vi "EOL Manual Sunroof Control.vi"(7 "remote sense enabled":bool, 9 "DO Task":refnum<k21>, 10 "station name":string, 11 "station idx":i32=4) -> ()   [LabVIEW 2018]
uses:
  02.Type Def's/EOL Analog Input Control.ctl
  02.Type Def's/All Motions.ctl
  05.UserVI's/type defs/EOL Part Setup.ctl
  02.Type Def's/All Communication Types.ctl
  05.UserVI's/type defs/Communication with Motors.ctl
  05.UserVI's/type defs/RAP Signal Control.ctl
  05.UserVI's/type defs/EOL Motor Type.ctl
  02.Type Def's/All Switch Configuration Cluster.ctl
  05.UserVI's/type defs/EOL Global Digital Output Control.ctl
  05.UserVI's/type defs/EOL Global Digital Output Cluster Control.ctl
panel:
  out "Part Infos":T1[](array[typedef])
  in  "Exit":bool
  in  "Tab Control 3":enum32{"Select Program", "Sunroof Operation"}(tab)=enum."Sunroof Operation"
  in  "Part Type Selected":bool
  in  "Part Type":u16(ring) items=["CD701", "NU2", "A07", "B41", "B26", "B30", "J4U"]
  in  "sunroof 4":bool
  in  "sunroof 3":bool
  in  "sunroof 2":bool
  in  "sunroof":bool
  in  "Ignition":bool
  in  "Power":bool
  in  "Switch Output":bool
  out "Audit Graph":sgl[][](graph)
  in  "Analog Control":T6=enum."Motor Voltage"
  in  "Analog Control 2":T6=enum."Motor Current"
  in  "Analog Control 3":T6=enum."Switch A"
  in  "Color Box 10":u32(colorbox)=16860
  in  "Color Box 11":u32(colorbox)=16711680
  in  "Color Box 12":u32(colorbox)
  in  "Current Motion":T7=enum."Glass Slide Open"
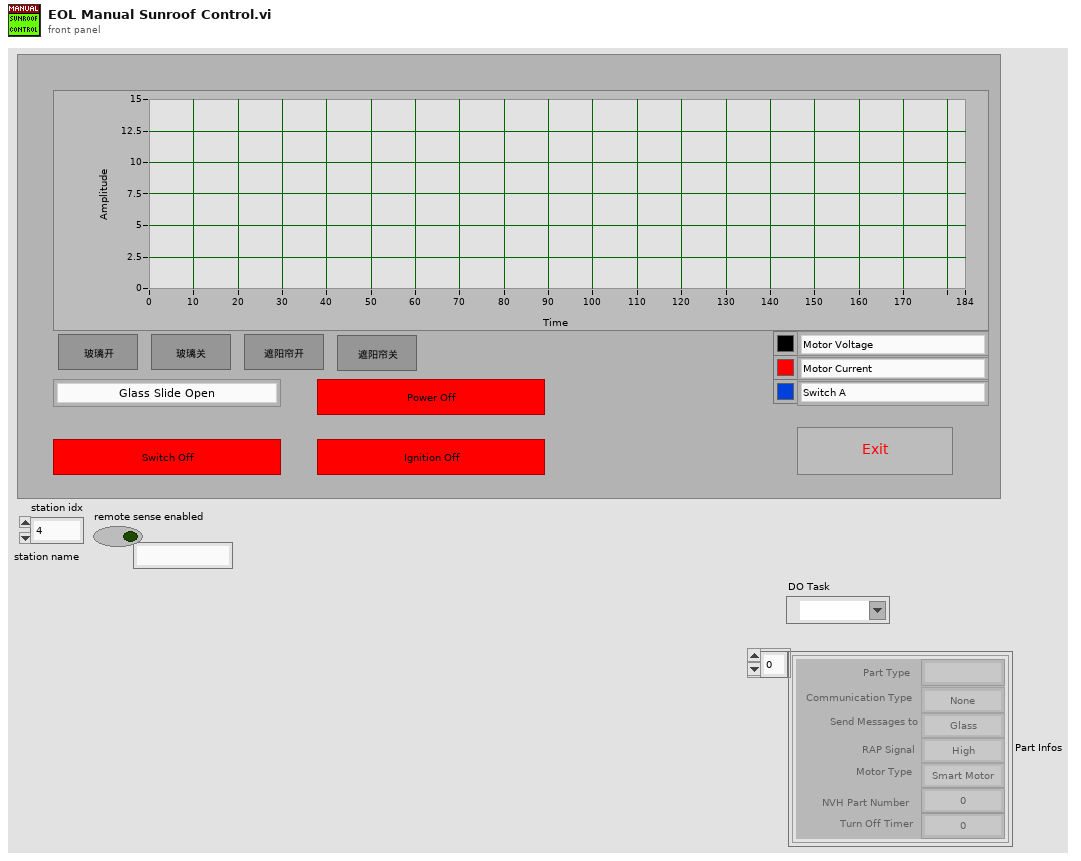
[diagram p1: front panel]
types:
  T1 = typedef "EOL Part Setup.ctl" = cluster{"Communication Type":T2, "Send Messages to":T3, "RAP Signal":T4, "Motor Type":T5, "NVH Part Number":u16, "Turn Off Timer":u16, "Part Type":string}
  T2 = typedef "All Communication Types.ctl" = enum16{"None", "CAN", "RS 232", "RS 232 LIN", "GM LIN", "SnT LIN", "K Line", "Robel CAN", "P42M-Continental", "Inalfa SCU LIN", "Spare 3"}
  T3 = typedef "Communication with Motors.ctl" = enum16{"Glass", "Rollo", "Both"}
  T4 = typedef "RAP Signal Control.ctl" = enum16{"High", "Low", "None"}
  T5 = typedef "EOL Motor Type.ctl" = enum16{"Smart Motor", "Sensor Motor"}
  T6 = typedef "EOL Analog Input Control.ctl" = enum16{"SW PS  Volage", "Switch A", "Switch B", "Switch C", "Motor Voltage", "Motor Current", "ATS"}
  T7 = typedef "All Motions.ctl" = enum16{"Glass Teach", "Glass Slide Open", "Glass Slide Close", "Glass Vent Open", "Glass Vent Close", "Sunshade Teach", "Sunshade Open", "Sunshade Close", "Idle", "Sunshade Open 2", "Sunshade Close 2", "Glass Slide Open Sunshade Open", "Glass Slide Open Sunshade Close", "Glass Slide Close Sunshade Open", "Glass Slide Close Sunshade Close", "Glass Vent Open Sunshade Open", "Glass Vent Open Sunshade Close", "Glass Vent Close Sunshade Open", "Glass Vent Close Sunshade Close", "Express Glass Slide Open", "Express Glass Slide Close", "Express Glass Vent Open", "Express Glass Vent Close", "Express Sunshade Open", "Express Sunshade Close", "Express Sunshade Open 2", "Express Sunshade Close 2", "Express Glass Slide Open Sunshade Open", "Express Glass Slide Open Sunshade Close", "Express Glass Slide Close Sunshade Open", "Express Glass Slide Close Sunshade Close", "Express Glass Vent Open Sunshade Open", "Express Glass Vent Open Sunshade Close", "Express Glass Vent Close Sunshade Open", "Express Glass Vent Close Sunshade Close", "Goto Position Glass", "Goto Position Sunshade", "Sunshade Teach 2"}
  T8 = typedef "All Switch Configuration Cluster.ctl" = cluster{"All Motions":T7, "A":bool[], "B":bool[], "C":bool[], "D":bool[], "A activation time (ms)":u32, "B activation time (ms)":u32, "C activation time (ms)":u32}
  T9 = cluster{"Part Type":string, "Switch Configuration":T8[]}
  T10 = enum16{"Init", "Write", "Write All", "Clear All", "Stop", "Read"}
  T11 = typedef "EOL Global Digital Output Control.ctl" = enum16{"Battery", "IGN High", "IGN Low", "LIN", "CAN", "Switch 1", "Switch 2", "Switch 3", "Switch 4", "Switch 5", "Switch 6", "Glass Analog Switch 1", "Glass Analog Switch 2", "Glass Analog Switch 3", "Glass Analog Switch 4", "Sunshade Analog Switch 1", "Sunshade Analog Switch 2", "Sunshade Analog Switch 3", "Sunshade Analog Switch 4", "Glass Motor Relay 1", "Glass Motor Relay 2", "Sunshade Motor Relay 1", "Sunshade Motor Relay 2"}
  T12 = typedef "EOL Global Digital Output Cluster Control.ctl" = cluster{"Status":bool, "Global DO Ch":T11}
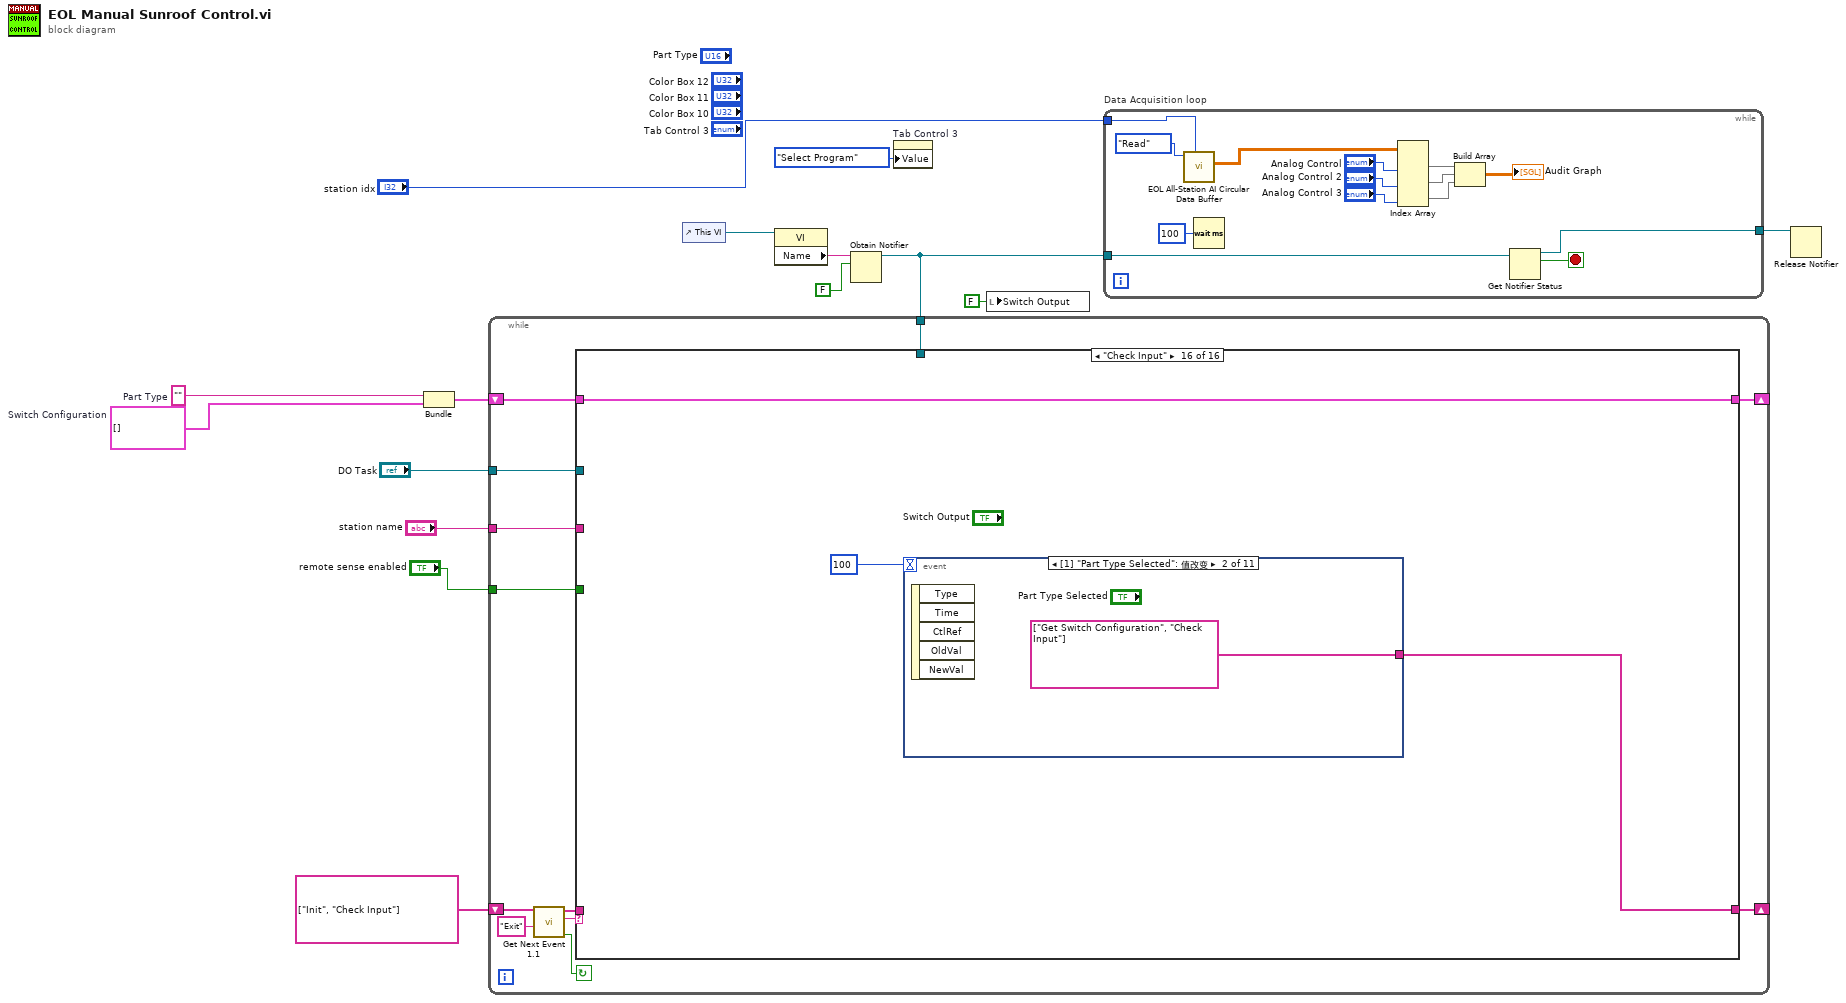
[diagram p0: block diagram]
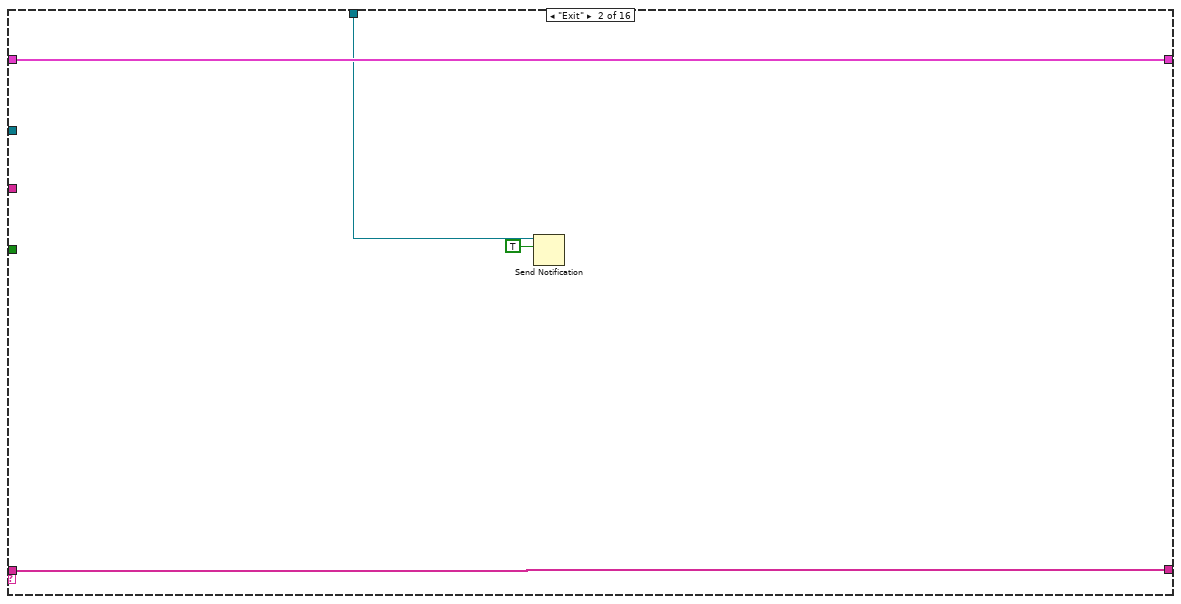
[diagram p3: hidden frame]
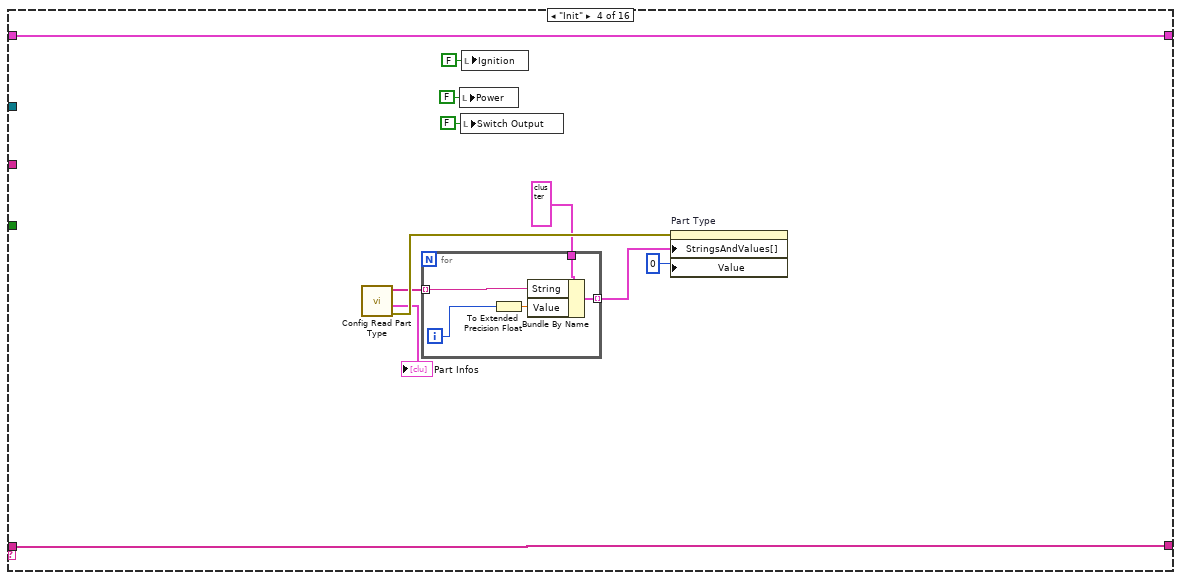
[diagram p5: hidden frame]
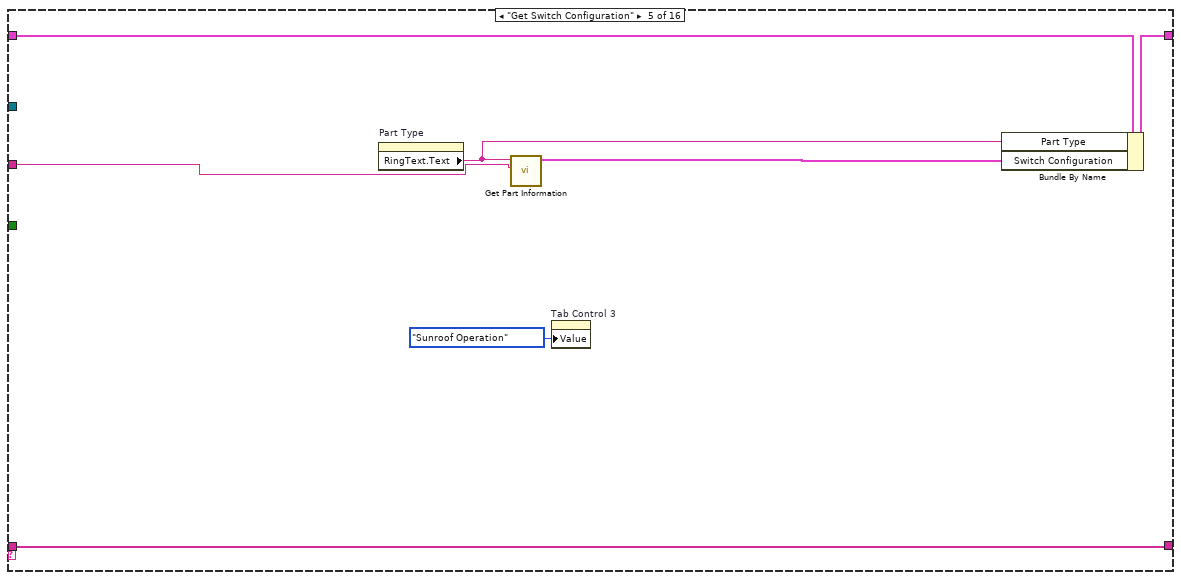
[diagram p6: hidden frame]
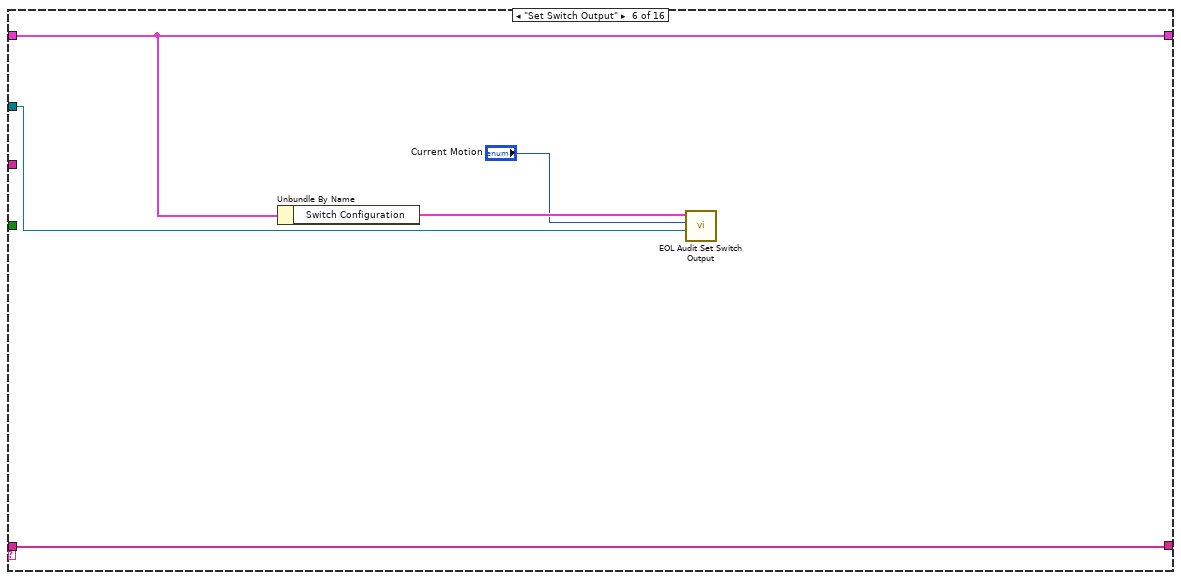
[diagram p7: hidden frame]
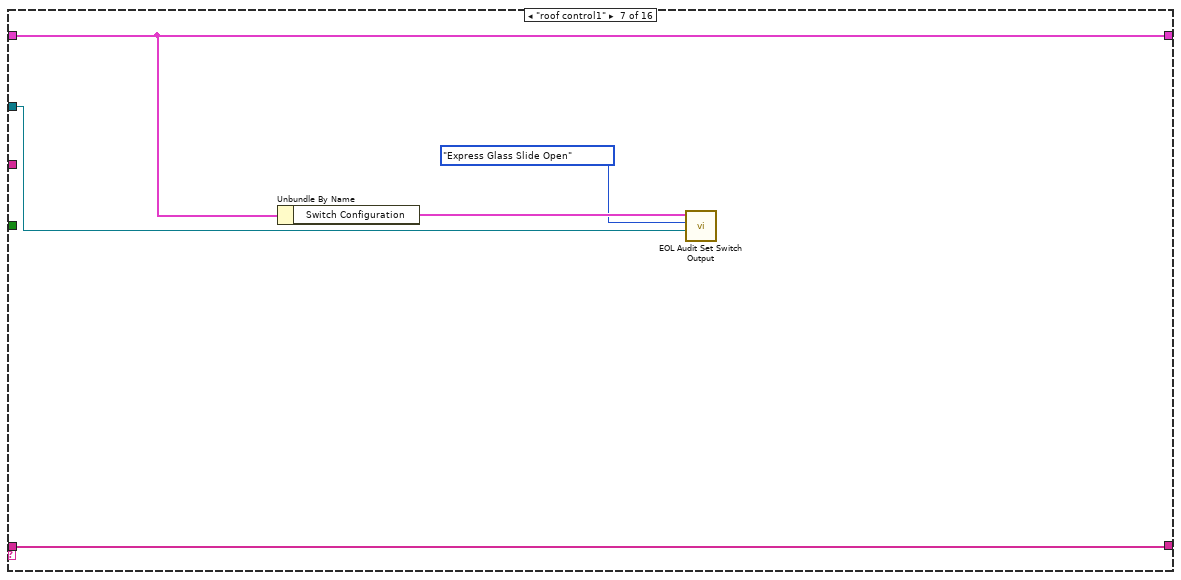
[diagram p8: hidden frame]
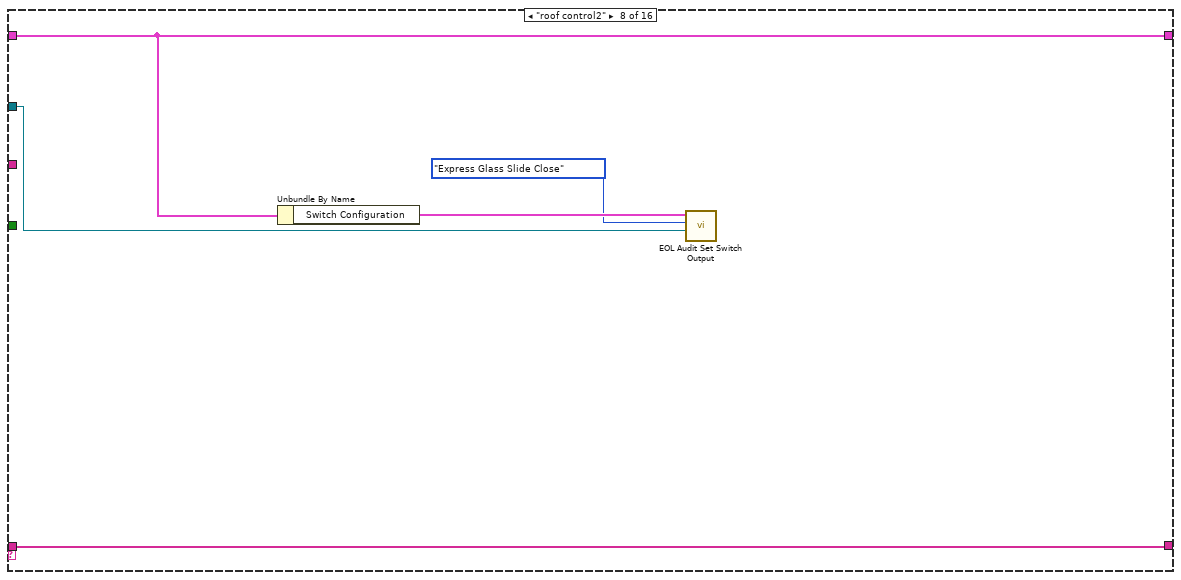
[diagram p9: hidden frame]
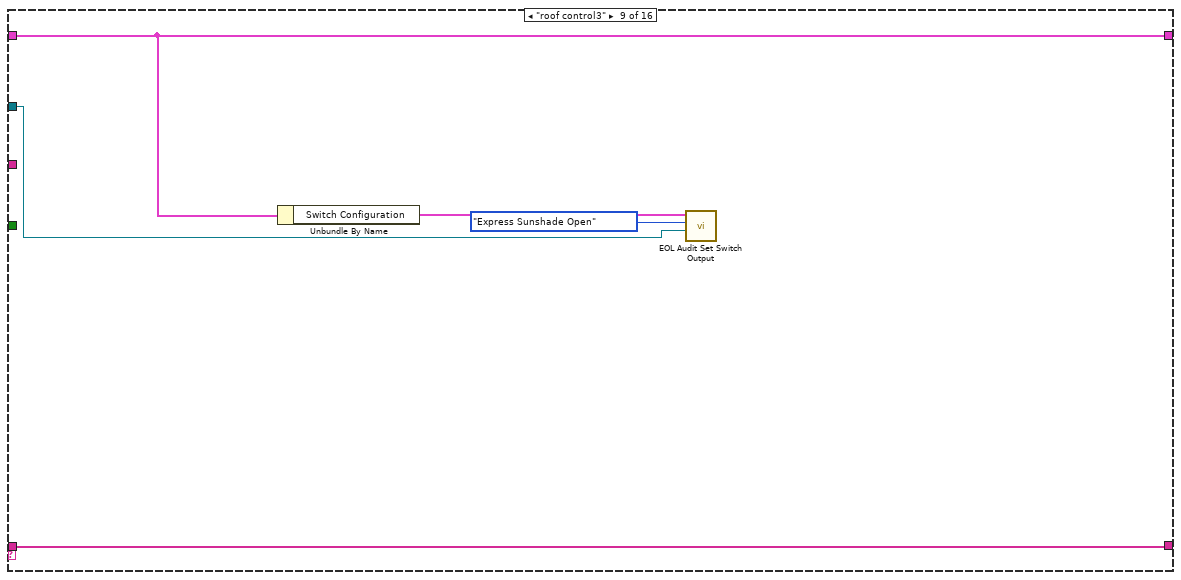
[diagram p10: hidden frame]
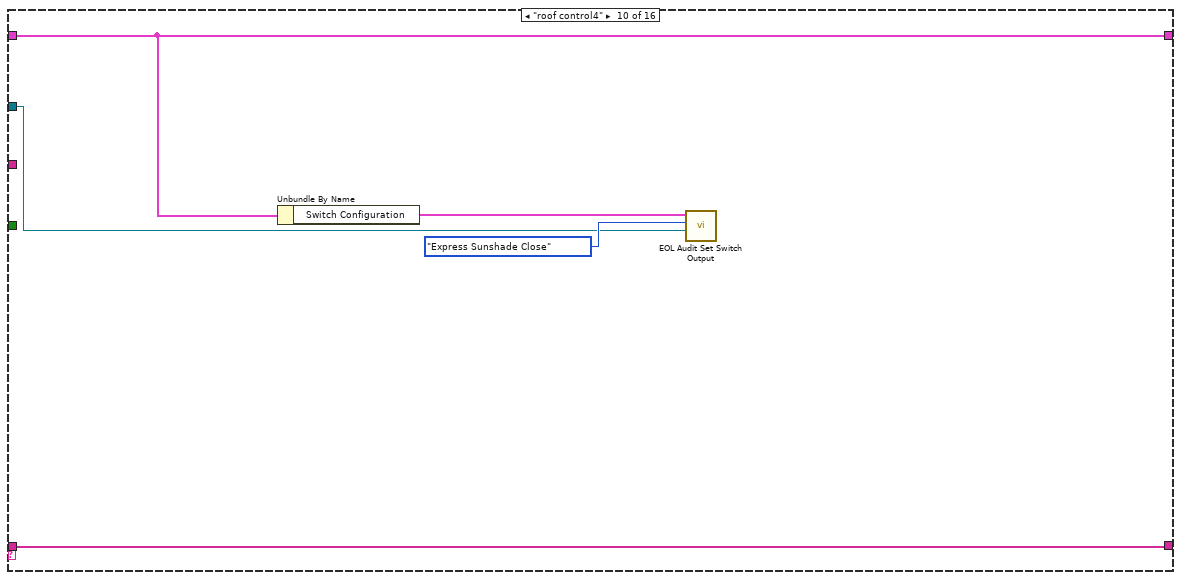
[diagram p11: hidden frame]
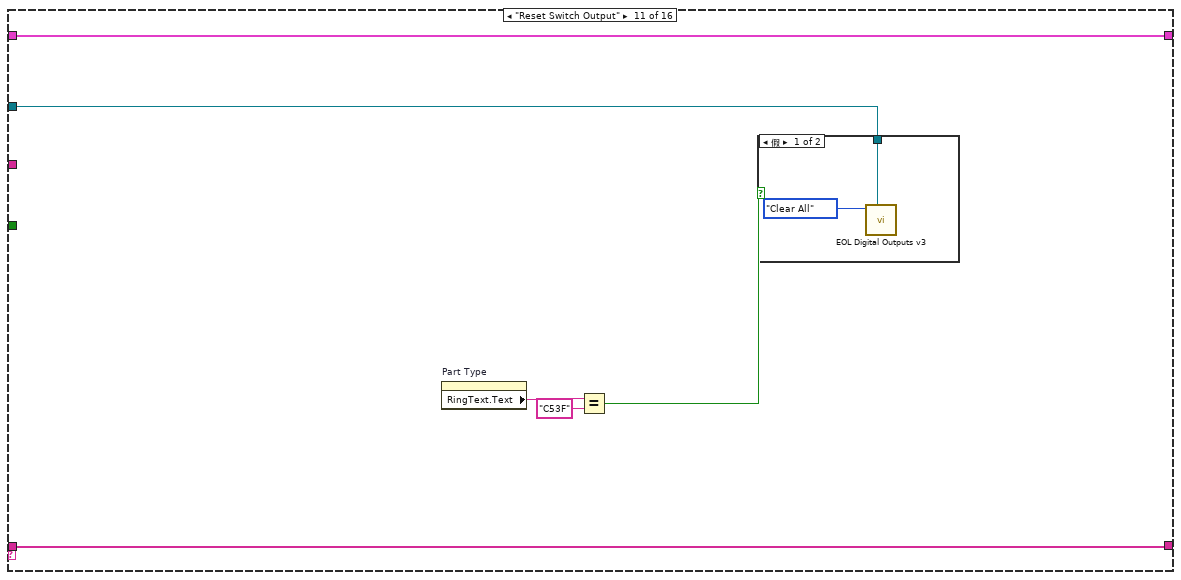
[diagram p12: hidden frame]
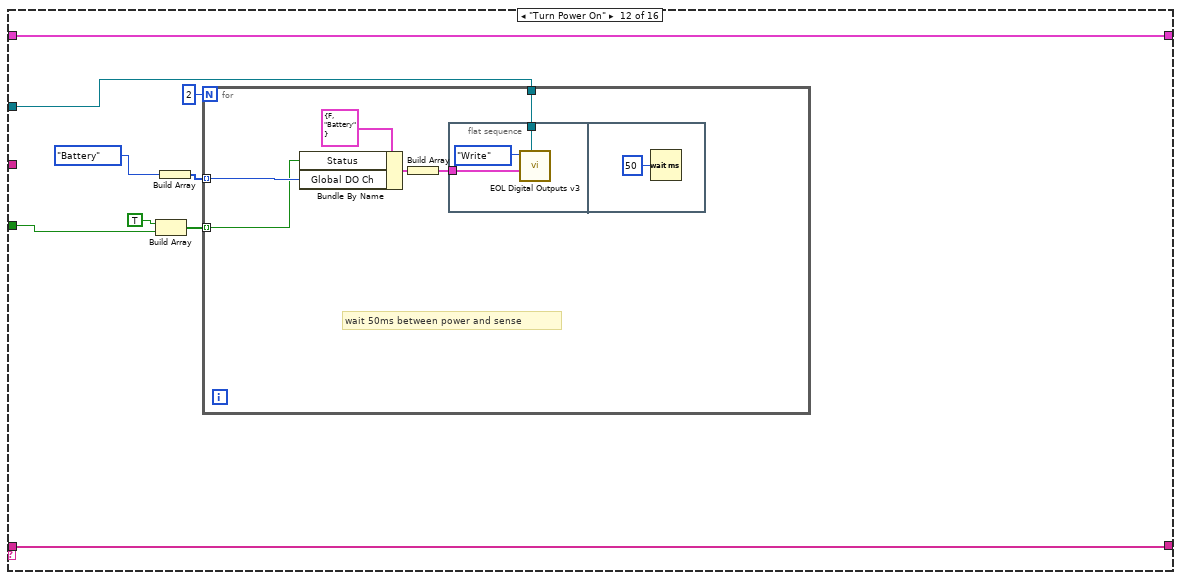
[diagram p14: hidden frame]
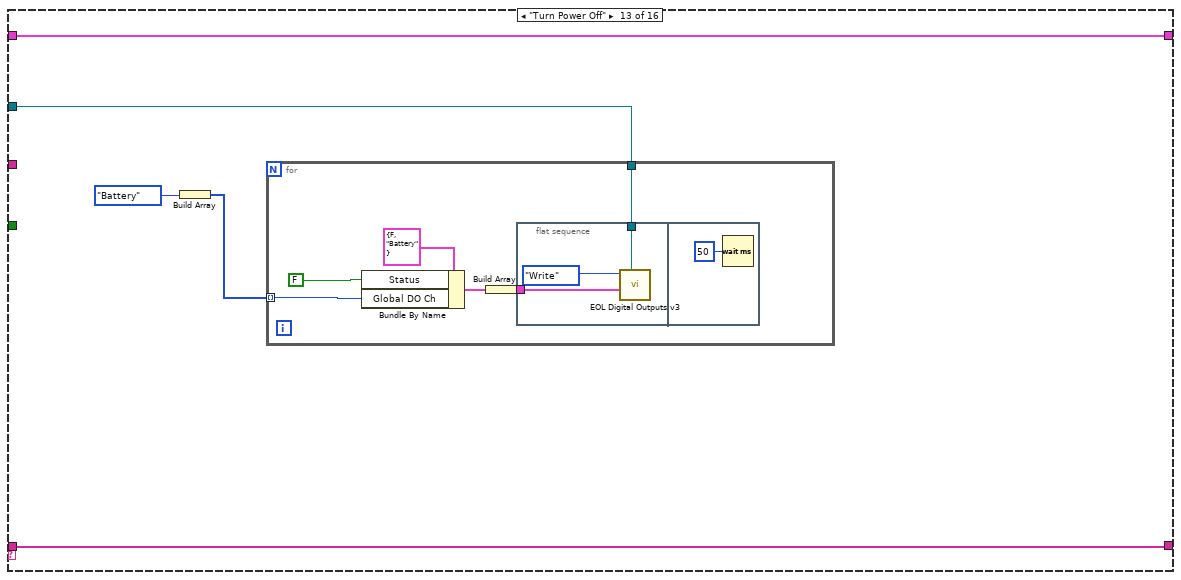
[diagram p15: hidden frame]
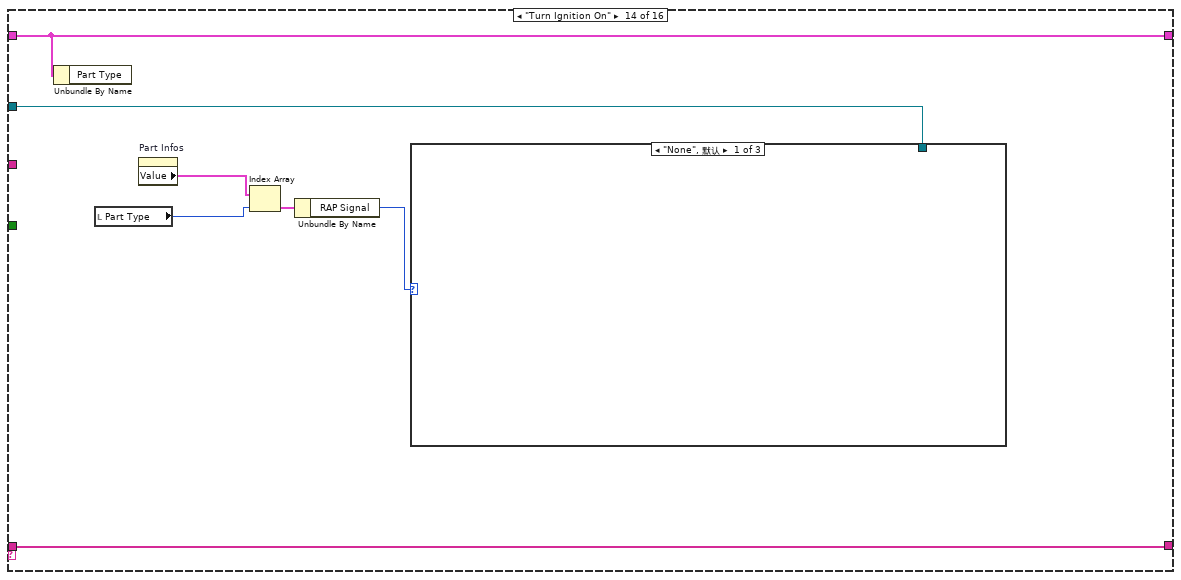
[diagram p16: hidden frame]
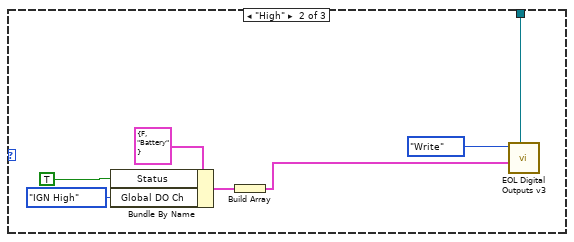
[diagram p17: hidden frame]
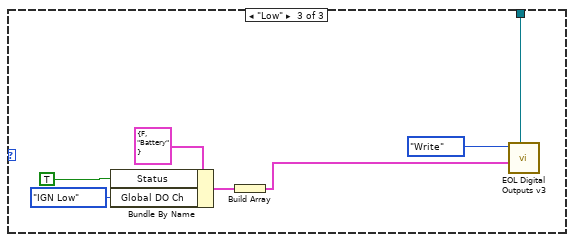
[diagram p18: hidden frame]
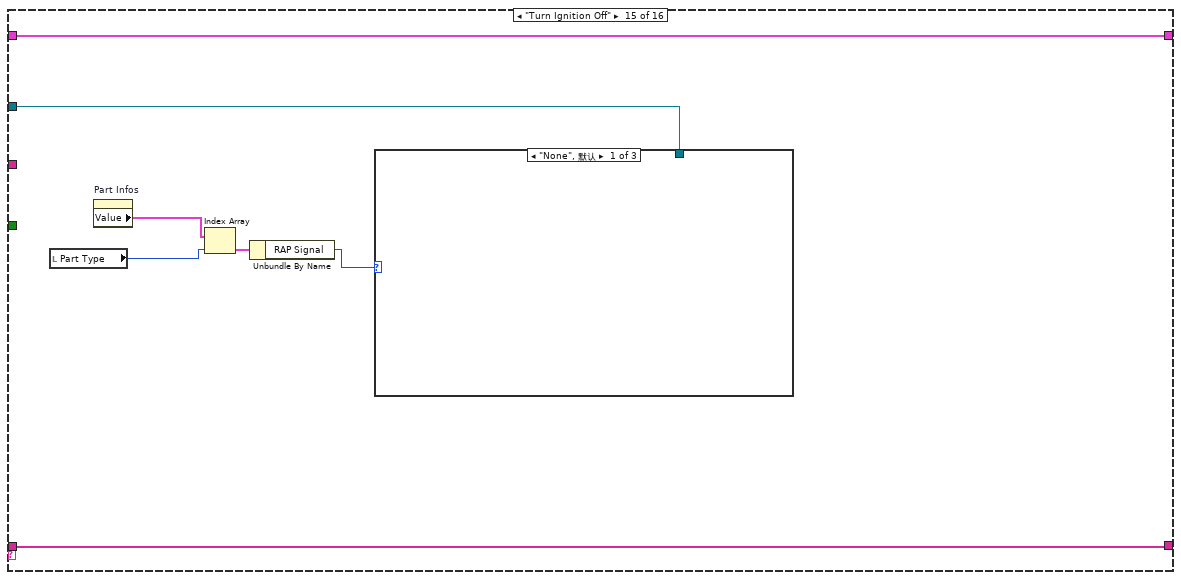
[diagram p19: hidden frame]
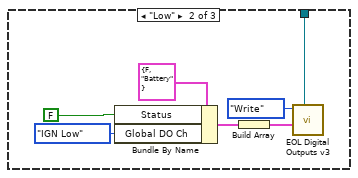
[diagram p20: hidden frame]
diagram:
  w12 = T8[] []  # Switch Configuration
  w14 = ""  # Part Type
  n1 = Bundle("Part Type"=w14, "Switch Configuration"=w12) -> (w15:T9)  [unwired: 1 in]
  n2 = control-ref of="This VI"() -> (w6:refnum<vi>)
  n3 = property class="VI"(reference=w6) -> ("Name"=w10:string)  [unwired: 1 in, 2 out]
  n4 = Obtain Notifier(name (unnamed)=w10, notification data type=FALSE) -> (notifier out=w8:refnum<notifier>)  [unwired: 2 in, 2 out]
  n5 = while {
    shift-right: [w25] -> _
    shift-left: string[] ["Init", "Check Input"] ("event queue out") -> [w24]
    shift-right: [w22] -> _
    shift-left: w15 -> [w23]
    tunnel: w8 -> [w19]
    tunnel: "station name" -> [w18]
    tunnel: "remote sense enabled" -> [w17]
    tunnel: "DO Task" -> [w16]
    stop <- w21 continue-if-true
    n6 = call "Get Next Event 1.1.vi"("Exit Event"="Exit", "event queue in"=w24) -> ("Condition (Exit:F)"=w21:bool, "next event"=w27:string, "event queue out"=w26:string[])  [unwired: 6 in, 1 out]
    n7 = case shown="\"Check Input\"" w27 {
      tunnel: w26 -> [w29 w33 w34 w46 w58 w63 w68 w73 w78 w83 w89 w99 w114 w132 w152 _]
      tunnel: [w29 w33 w34 w46 w58 w63 w68 w73 w78 w83 w89 w99 w114 w132 w152 w169] -> w25
      tunnel: w23 -> [w28 w32 w35 w45 w57 w62 w67 w72 w77 w82 w88 w100 w115 w130 w153 w170]
      tunnel: [w28 w32 w35 w45 w56 w62 w67 w72 w77 w82 w88 w100 w115 w130 w153 w170] -> w22
      tunnel: w19 -> [_ w31 _ _ _ _ _ _ _ _ _ _ _ _ _ _]
      tunnel: w18 -> [_ _ _ _ w52 _ _ _ _ _ _ _ _ _ _ _]
      tunnel: w17 -> [_ _ _ _ _ _ _ _ _ _ _ w96 _ _ _ _]
      tunnel: w16 -> [_ _ _ _ _ w59 w64 w69 w74 w79 w84 w92 w111 w131 w151 _]
      frame "Error", Default {
      }
      frame "Exit" {
        n8 = Send Notification(notification=TRUE, notifier=w31) -> ()  [unwired: 1 in, 2 out]
      }
      frame "Analog Data" {
      }
      frame "Init" {
        n9 = call "Config Read Part Type.vi"() -> ("Error Out"=w44:errorcluster, "Part Infos"=→"Part Infos":T1[], "Part Types"=w40:string[])  [unwired: 9 in]
        n10 = for {
          tunnel: cluster{"String":string, "Value":ext} {"String"="", "Value"=0.0} -> [w51]
          tunnel: w40 -> [w49] mode=indexing
          tunnel: [w48] -> w41 mode=indexing
          i -> [w47]
          n11 = To Extended Precision Float(1:w47) -> (0:w50:ext)
          n12 = Bundle By Name(cluster=w51, "String"=w49, "Value"=w50) -> (w48:cluster{"String":string, "Value":ext})
        }
        n13 = local write "Power"(FALSE ("Power")) -> ()
        n14 = local write "Switch Output"(FALSE ("Switch Output")) -> ()
        n15 = local write "Ignition"(FALSE ("Ignition")) -> ()
        n16 = property on="Part Type" class="Ring (strict)"(error in=w44, "StringsAndValues[]"=w41, "Value"=u16 0) -> ()  [unwired: 1 in, 2 out]
      }
      frame "Get Switch Configuration" {
        n17 = property on="Part Type" class="Ring (strict)"() -> ("RingText.Text"=w54:string)  [unwired: 2 in, 2 out]
        n18 = call "Get Part Information.vi"("station name"=w52, "Part Type"=w54) -> ("Switch Configuration"=w55:T8[])  [unwired: 1 in, 8 out]
        n19 = property on="Tab Control 3" class="TabCtl (strict)"("Value"=enum32{"Select Program", "Sunroof Operation"}."Sunroof Operation" ("Tab Control 3")) -> ()  [unwired: 2 in, 2 out]
        n20 = Bundle By Name(cluster=w57, "Part Type"=w54, "Switch Configuration"=w55) -> (w56:T9)
      }
      frame "Set Switch Output" {
        n21 = Unbundle By Name(w62) -> ("Switch Configuration"=w61:T8[])
        n22 = call "EOL Audit Set Switch Output.vi"("task/channels in"=w59, "Current Motion"="Current Motion", "Switch Output Array"=w61) -> ()  [unwired: 6 in, 3 out]
      }
      frame "roof control1" {
        n23 = Unbundle By Name(w67) -> ("Switch Configuration"=w66:T8[])
        n24 = call "EOL Audit Set Switch Output.vi"("task/channels in"=w64, "Current Motion"=All_Motions."Express Glass Slide Open", "Switch Output Array"=w66) -> ()  [unwired: 6 in, 3 out]
      }
      frame "roof control2" {
        n25 = Unbundle By Name(w72) -> ("Switch Configuration"=w71:T8[])
        n26 = call "EOL Audit Set Switch Output.vi"("task/channels in"=w69, "Current Motion"=All_Motions."Express Glass Slide Close", "Switch Output Array"=w71) -> ()  [unwired: 6 in, 3 out]
      }
      frame "roof control3" {
        n27 = Unbundle By Name(w77) -> ("Switch Configuration"=w76:T8[])
        n28 = call "EOL Audit Set Switch Output.vi"("task/channels in"=w74, "Current Motion"=All_Motions."Express Sunshade Open", "Switch Output Array"=w76) -> ()  [unwired: 6 in, 3 out]
      }
      frame "roof control4" {
        n29 = Unbundle By Name(w82) -> ("Switch Configuration"=w81:T8[])
        n30 = call "EOL Audit Set Switch Output.vi"("task/channels in"=w79, "Current Motion"=All_Motions."Express Sunshade Close", "Switch Output Array"=w81) -> ()  [unwired: 6 in, 3 out]
      }
      frame "Reset Switch Output" {
        n31 = property on="Part Type" class="Ring (strict)"() -> ("RingText.Text"=w87:string)  [unwired: 2 in, 2 out]
        n32 = Equal?(x=w87, y="C53F") -> (x = y?=w85:bool)
        n33 = case shown="假" w85 {
          tunnel: w84 -> [w90 _]
          frame False {
            n34 = call "EOL Digital Outputs v3.vi"("task/channels in"=w90, "Mode"=T10."Clear All") -> ()  [unwired: 8 in, 2 out]
          }
          frame True {
          }
        }
      }
      frame "Turn Power On" {
        n35 = Build Array(TRUE ("Status"), w96) -> (w94:bool[])
        n36 = Build Array(EOL_Global_Digital_Output_Control."Battery" ("Global DO Ch")) -> (w97:T11[])
        n37 = for {
          N: 2 -> [_]
          tunnel: w97 -> [w104] mode=indexing
          tunnel: w94 -> [w102] mode=indexing
          tunnel: w92 -> [w101]
          # "wait 50ms between power and sense"
          n38 = Bundle By Name(cluster=T12 {"Status"=FALSE, "Global DO Ch"=enum."Battery"} ("Cluster"), "Status"=w102, "Global DO Ch"=w104) -> (w105:T12)
          n39 = Build Array(w105) -> (w103:T12[])
          n40 = flat-sequence {
            tunnel: w103 -> [w108]
            tunnel: w101 -> [w107]
            frame #0 {
              n41 = call "EOL Digital Outputs v3.vi"("task/channels in"=w107, "DO Status"=w108, "Mode"=T10."Write") -> ()  [unwired: 7 in, 2 out]
            }
            frame #1 {
              n42 = Wait (ms)(milliseconds to wait=u32 50) -> ()  [unwired: 1 out]
            }
          }
        }
      }
      frame "Turn Power Off" {
        n43 = Build Array(EOL_Global_Digital_Output_Control."Battery" ("Global DO Ch")) -> (w113:T11[])
        n44 = for {
          tunnel: w113 -> [w118] mode=indexing
          tunnel: w111 -> [w116]
          n45 = Bundle By Name(cluster=T12 {"Status"=FALSE, "Global DO Ch"=enum."Battery"} ("Cluster"), "Status"=FALSE, "Global DO Ch"=w118) -> (w119:T12)
          n46 = Build Array(w119) -> (w117:T12[])
          n47 = flat-sequence {
            tunnel: w117 -> [w123]
            tunnel: w116 -> [w122]
            frame #0 {
              n48 = call "EOL Digital Outputs v3.vi"("task/channels in"=w122, "DO Status"=w123, "Mode"=T10."Write") -> ()  [unwired: 7 in, 2 out]
            }
            frame #1 {
              n49 = Wait (ms)(milliseconds to wait=u32 50) -> ()  [unwired: 1 out]
            }
          }
        }
      }
      frame "Turn Ignition On" {
        n50 = Unbundle By Name(w130) -> ()  [unwired: 1 out]
        n51 = local read "Part Type"() -> (w128:u16)
        n52 = property on="Part Infos" class="Arr (strict)"() -> ("Value"=w129:T1[])  [unwired: 2 in, 2 out]
        n53 = Index Array(array=w129, index=w128) -> (element=w127:T1)
        n54 = Unbundle By Name(w127) -> ("RAP Signal"=w126:T4)
        n55 = case shown="\"None\", 默认" w126 {
          tunnel: w131 -> [_ w133 w140]
          frame "None", Default {
          }
          frame "High" {
            n56 = Bundle By Name(cluster=T12 {"Status"=FALSE, "Global DO Ch"=enum."Battery"} ("Cluster"), "Status"=TRUE, "Global DO Ch"=EOL_Global_Digital_Output_Control."IGN High") -> (w136:T12)
            n57 = Build Array(w136) -> (w135:T12[])
            n58 = call "EOL Digital Outputs v3.vi"("task/channels in"=w133, "DO Status"=w135, "Mode"=T10."Write") -> ()  [unwired: 7 in, 2 out]
          }
          frame "Low" {
            n59 = Bundle By Name(cluster=T12 {"Status"=FALSE, "Global DO Ch"=enum."Battery"} ("Cluster"), "Status"=TRUE, "Global DO Ch"=EOL_Global_Digital_Output_Control."IGN Low") -> (w143:T12)
            n60 = Build Array(w143) -> (w142:T12[])
            n61 = call "EOL Digital Outputs v3.vi"("task/channels in"=w140, "DO Status"=w142, "Mode"=T10."Write") -> ()  [unwired: 7 in, 2 out]
          }
        }
      }
      frame "Turn Ignition Off" {
        n62 = local read "Part Type"() -> (w149:u16)
        n63 = property on="Part Infos" class="Arr (strict)"() -> ("Value"=w150:T1[])  [unwired: 2 in, 2 out]
        n64 = Index Array(array=w150, index=w149) -> (element=w148:T1)
        n65 = Unbundle By Name(w148) -> ("RAP Signal"=w147:T4)
        n66 = case shown="\"None\", 默认" w147 {
          tunnel: w151 -> [_ w154 w161]
          frame "None", Default {
          }
          frame "Low" {
            n67 = Bundle By Name(cluster=T12 {"Status"=FALSE, "Global DO Ch"=enum."Battery"} ("Cluster"), "Status"=FALSE, "Global DO Ch"=EOL_Global_Digital_Output_Control."IGN Low") -> (w157:T12)
            n68 = Build Array(w157) -> (w156:T12[])
            n69 = call "EOL Digital Outputs v3.vi"("task/channels in"=w154, "DO Status"=w156, "Mode"=T10."Write") -> ()  [unwired: 7 in, 2 out]
          }
          frame "High" {
            n70 = Bundle By Name(cluster=T12 {"Status"=FALSE, "Global DO Ch"=enum."Battery"} ("Cluster"), "Status"=FALSE, "Global DO Ch"=EOL_Global_Digital_Output_Control."IGN Low") -> (w164:T12)
            n71 = Build Array(w164) -> (w163:T12[])
            n72 = call "EOL Digital Outputs v3.vi"("task/channels in"=w161, "DO Status"=w163, "Mode"=T10."Write") -> ()  [unwired: 7 in, 2 out]
          }
        }
      }
      frame "Check Input" {
        n73 = event shown="[1] \"Part Type Selected\": 值改变" {
          selector: _ -> [_ _ _ _ _ _ _ _ _ _ _]
          dyn-events: _ -> [_ _ _ _ _ _ _ _ _ _ _]
          timeout: 100 -> [_ _ _ _ _ _ _ _ _ _ _]
          tunnel: [string[] ["Check Input"] ("event queue out") string[] ["Get Switch Configuration", "Check Input"] ("event queue out") string[] ["Set Switch Output", "Check Input"] ("event queue out") string[] ["Reset Switch Output", "Check Input"] ("event queue out") w176 w180 string[] ["Turn Ignition On", "Turn Power On", "roof control1", "Check Input"] ("event queue out") string[] ["Turn Ignition On", "Turn Power On", "roof control2", "Check Input"] ("event queue out") string[] ["Turn Ignition On", "Turn Power On", "roof control3", "Check Input"] ("event queue out") string[] ["Turn Ignition On", "Turn Power On", "roof control4", "Check Input"] ("event queue out") string[] ["Reset Switch Output", "Exit"] ("event queue out")] -> w169
          event Timeout {
            n74 = event-data() -> ()  [unwired: 1 in, 2 out]
          }
          event "Part Type Selected": Value Change {
            n75 = event-data() -> ()  [unwired: 1 in, 5 out]
          }
          event "Switch Output": Mouse Down {
            n76 = event-data() -> ()  [unwired: 1 in, 7 out]
          }
          event "Switch Output": Mouse Up; "Switch Output": Mouse Leave {
            n77 = event-data() -> ()  [unwired: 1 in, 3 out]
          }
          event "Power": Value Change {
            n78 = event-data() -> ("NewVal"=w175:bool)  [unwired: 1 in, 4 out]
            n79 = case shown="真" w175 {
              tunnel: [string[] ["Turn Power On", "Check Input"] ("event queue out") string[] ["Turn Power Off", "Check Input"] ("event queue out")] -> w176
              frame True {
              }
              frame False {
              }
            }
          }
          event "Ignition": Value Change {
            n80 = event-data() -> ("NewVal"=w179:bool)  [unwired: 1 in, 4 out]
            n81 = case shown="真" w179 {
              tunnel: [string[] ["Turn Ignition On", "Check Input"] ("event queue out") string[] ["Turn Ignition Off", "Check Input"] ("event queue out")] -> w180
              frame True {
              }
              frame False {
              }
            }
          }
          event "sunroof": Value Change {
            n82 = event-data() -> ()  [unwired: 1 in, 6 out]
          }
          event "sunroof 2": Value Change {
            n83 = event-data() -> ()  [unwired: 1 in, 6 out]
          }
          event "sunroof 3": Value Change {
            n84 = event-data() -> ()  [unwired: 1 in, 6 out]
          }
          event "sunroof 4": Value Change {
            n85 = event-data() -> ()  [unwired: 1 in, 6 out]
          }
          event "Exit": Value Change {
            n86 = event-data() -> ()  [unwired: 1 in, 5 out]
          }
        }
      }
    }
  }
  n87 = property on="Tab Control 3" class="TabCtl (strict)"("Value"=enum32{"Select Program", "Sunroof Operation"}."Select Program" ("Tab Control 3")) -> ()  [unwired: 2 in, 2 out]
  n88 = local write "Switch Output"(FALSE ("Switch Output")) -> ()
  n89 = while "Data Acquisition loop" {
    tunnel: w8 -> [w196]
    tunnel: [w194] -> w7
    tunnel: "station idx" -> [w191]
    stop <- w195 stop-if-true
    n90 = call "EOL All-Station AI Circular Data Buffer.vi"("station idx"=w191, "Mode"=enum16{"Initialize", "Read", "Write"}."Read") -> ("Data Read (Samp-Ro, Ch-Col)"=w192:sgl[][])  [unwired: 9 in]
    n91 = Wait (ms)(milliseconds to wait=u32 100) -> ()  [unwired: 1 out]
    n92 = Index Array(array=w192, index (col) #1="Analog Control", index (col) #2="Analog Control 2", index (col) #3="Analog Control 3") -> (element #1=w201:sgl[], element #2=w200:sgl[], element #3=w199:sgl[])  [unwired: 3 in]
    n93 = Build Array(w201, w200, w199) -> (→"Audit Graph":sgl[][])
    n94 = Get Notifier Status(notifier=w196) -> (notifier out=w194:refnum<notifier>, current notification=w195:bool)  [unwired: 1 in, 3 out]
  }
  n95 = Release Notifier(notifier=w7) -> ()  [unwired: 2 in, 3 out]
